vi "Read VISA resource name.vi"(11 "Instrumento in":refnum<class "Instrumento.lvclass">) -> (2 "VISA resource name":refnum<visa-resource-name>, 3 "Instrumento out":refnum<class "Instrumento.lvclass">)   [LabVIEW 2020, in "Instrumento.lvclass"]
uses:
  Instrumento.lvclass
  Instrumento.lvclass/Instrumento.ctl
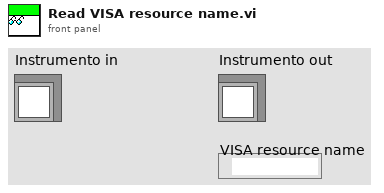
[diagram p1: front panel]
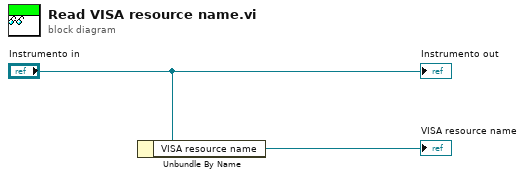
[diagram p0: block diagram]
diagram:
  n1 = Unbundle By Name("Instrumento in") -> ("VISA resource name"=→"VISA resource name":refnum<visa-resource-name>)
  "Instrumento out" <- "Instrumento in"
